vi "[RT] Finite Acq.vi"() -> ()   [LabVIEW 2015]
doc: "The finite acquisition mode tells the FPGA to acquire a certain number of samples and then terminate the acquisition. In this acquisition mode, the rwfm_ConfigTiming VI calls rwfm_BufferConfig.vi and sets the host application's data buffer size equal to the number of points in the finite acquisition."
uses:
  <vilib>/NI/cRIO Wfm/ChannelConfig.ctl
  <vilib>/FPGAPlugInAG/sbRIO-9607/niLvFpga_Open_sbRIO-9607.vi
  <vilib>/rvi/interface/common/dynamic/niFpgaDynamicAddResources.vi
  <vilib>/FPGAPlugInAG/Dynamic/niLvFpga_Reset_Dynamic.vi
  <vilib>/FPGAPlugInAG/Dynamic/niLvFpga_Run_Dynamic.vi
  IFw_Addon/RT/ReadWaveform.vi
  <vilib>/FPGAPlugInAG/Dynamic/niLvFpga_Close_Dynamic.vi
  <vilib>/rvi/interface/nirviOpenFPGA/nirviOpenFPGA.xnode
  FPGA Bitfiles/WaveformLibraryI_FPGATarget2_[FPGA]SARAcqMain_U+qOsuK4w1s.lvbitx
  FPGA/[FPGA] SAR Acq Main.vi
  <vilib>/rvi/interface/nirviMethod/nirviMethod.xnode
  <vilib>/rvi/interface/nirviCloseFPGA/nirviCloseFPGA.xnode
  IFw_Addon/RT/WaveformTask.lvclass
  <vilib>/NI/cRIO Wfm/cRIO Wfm.lvlib
panel:
  in  "Sample Rate":u32=51200
  in  "Channel Info":T1=[{"Channel Name"="Mod1/ai0", "Sensitivity mV_EU"=1000.0, "EU"="V", "dB Ref EU"=1.0}, {"Channel Name"="Mod1/ai1", "Sensitivity mV_EU"=1000.0, "EU"="V", "dB Ref EU"=1.0}, {"Channel Name"="Mod1/ai2", "Sensitivity mV_EU"=1000.0, "EU"="V", "dB Ref EU"=1.0}] caption="Channel Name      Scale [mV/EU]        EU           dB Ref [EU]" {"dB Ref EU" format="%#.2p"; "Sensitivity mV_EU" format="%.2f"}
  out "Waveform Graph":waveform(sgl)[](graph)
  in  "Samps per Chan":i32=25600 caption="Samples per Channel"
  # "Sampling Info"
  # "Channel Info"
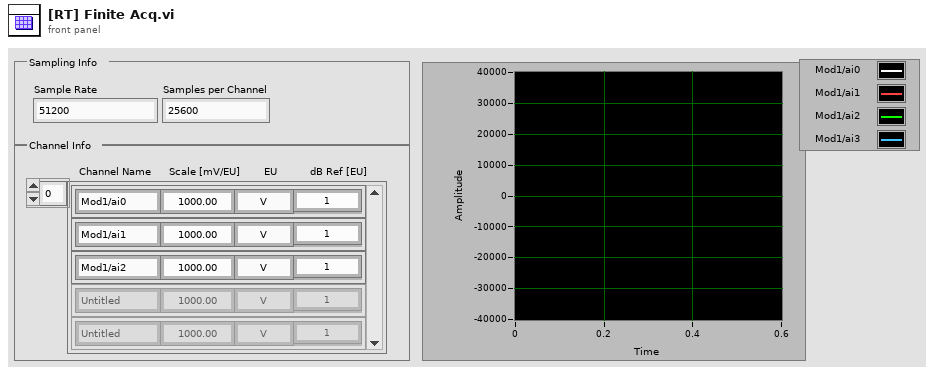
[diagram p1: front panel]
types:
  T1 = typedef "cRIO Wfm.lvlib/ChannelConfig.ctl" = cluster{"Channel Name":string, "Sensitivity mV_EU":dbl, "EU":string, "dB Ref EU":dbl}[]
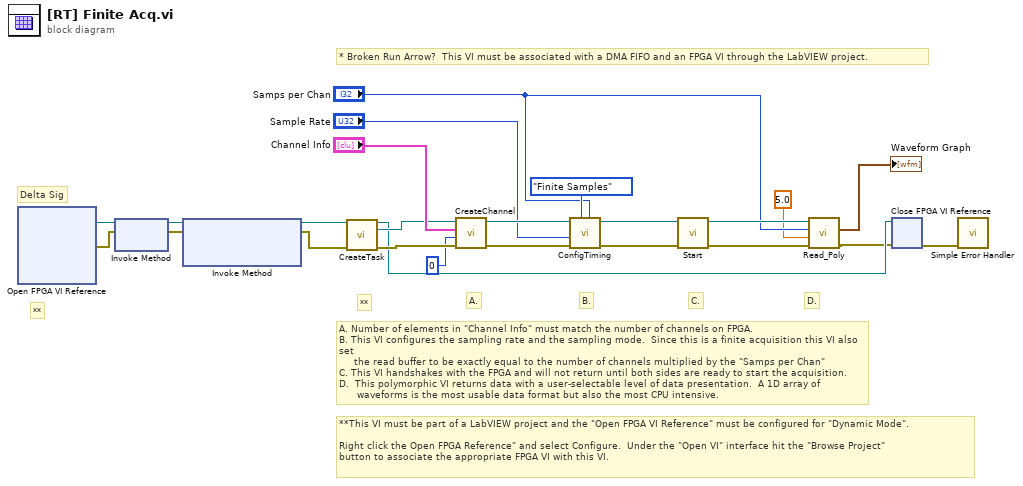
[diagram p0: block diagram]
diagram:
  # "Delta Sig"
  # "**"
  # "**This VI must be part of a LabVIEW project and the \"Open FPGA VI Reference\" must be configured for \"Dynamic Mode\".\n\nRight click the Open FPGA Reference\" and select Configure.  Under the \"Open VI\" interface hit the \"Browse Project\" \nbutton to associate the appropriate FPGA VI with this VI."
  # "* Broken Run Arrow?  This VI must be associated with a DMA FIFO and an FPGA VI through the LabVIEW project."
  # "A. Number of elements in \"Channel Info\" must match the number of channels on FPGA.\nB. This VI configures the sampling rate and the sampling mode.  Since this is a finite acquisition this VI also set  \n     the read buffer to be exactly equal to the number of channels multiplied by the \"Samps per Chan\"\nC. This VI handshakes with the FPGA and will not return until both sides are ready to start the acquisition.\nD.  This polymorphic VI returns data with a user-selectable level of data presentation.  A 1D array of     \n      waveforms is the most usable data format but also the most CPU intensive."
  # "**"
  # "D."
  # "C."
  # "B."
  # "A."
  n1 = xnode "Open FPGA VI Reference"() -> ("FPGA VI Reference Out"=w14:refnum<k20>, "error out"=w13:errorcluster)  [unwired: 2 in]
  n2 = xnode "Invoke Method"("FPGA VI Reference In"=w14, "error in"=w13) -> ("FPGA VI Reference Out"=w16:refnum<k20>, "error out"=w15:errorcluster)
  n3 = xnode "Invoke Method"("FPGA VI Reference In"=w16, "error in"=w15) -> ("FPGA VI Reference Out"=w12:refnum<k20>, "error out"=w11:errorcluster)  [unwired: 1 in]
  n4 = call "CreateTask.vi"("FPGA Ref in"=w12, "error in"=w11) -> ("FPGA Ref out"=w8:refnum<k20>, "Task out"=w9:refnum<class "WaveformTask.lvclass">, "error out"=w10:errorcluster)  [unwired: 11 in]
  n5 = call "CreateChannel.vi"("error in"=w10, "instance"=u8 0, "Channel Info"="Channel Info", "task in"=w9) -> ("error out"=w21:errorcluster, "Task out"=w22:refnum<class "WaveformTask.lvclass">)  [unwired: 6 in]
  n6 = call "ConfigTiming.vi"("Samples per Channel"="Samps per Chan", "Sample Mode"=enum16{"Finite Samples", "Continuous Samples"}."Finite Samples", "error in (no error)"=w21, "Sample Rate"="Sample Rate", "Task in"=w22) -> ("error out"=w19:errorcluster, "Task out"=w20:refnum<class "WaveformTask.lvclass">)  [unwired: 4 in, 1 out]
  n7 = call "Start.vi"("error in (no error)"=w19, "WaveformTask in"=w20) -> ("error out"=w5:errorcluster, "WaveformTask out"=w6:refnum<class "WaveformTask.lvclass">)  [unwired: 8 in]
  n8 = call-poly "Read_Poly.vi"("error in"=w5, "Timeout (s)"=5.0, "Samps Read per Chan"="Samps per Chan", "Task in"=w6) -> ("error out"=w4:errorcluster, "Waveforms"=→"Waveform Graph":waveform(sgl)[])  [unwired: 4 in, 2 out]
  n9 = xnode "Close FPGA VI Reference"("FPGA VI Reference In"=w8, "error in"=w4) -> ("error out"=w23:errorcluster)
  n10 = call <vilib>:"Simple Error Handler.vi"("error in (no error)"=w23) -> ()  [unwired: 1 in, 8 out]
